vi "populate listbox with logged channels.vi"(7 "MulticolumnListbox in":refnum<vi>, 8 "error in":errorcluster, 11 "Item Ref in":T1 format="%.0x") -> (0 "error out":errorcluster, 2 "logged channel shortnames":string[](array[string]), 3 "logged channel refs":T1[](array[typedef]) format="%.0x")   [LabVIEW 2026, in "Nominal Core Streaming System Explorer.lvlib"]
uses:
  Nominal Core Streaming System Explorer.lvlib
  <vilib>/NI VeriStand/Custom Device API/Custom Device Item Ref.ctl
  <vilib>/NI VeriStand/Custom Device API/Custom Device API.lvlib
  Shared/Nominal Core Streaming Shared.lvlib
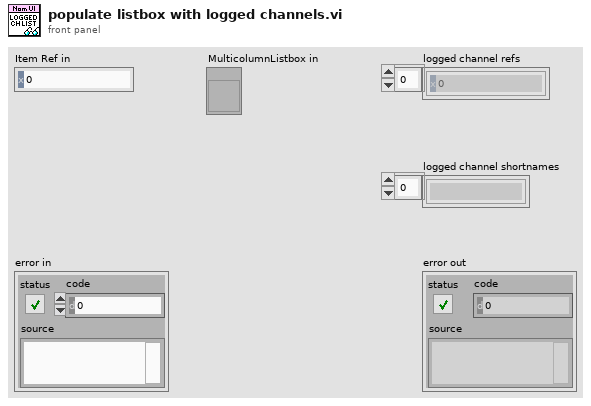
[diagram p1: front panel]
types:
  T1 = typedef "Custom Device API.lvlib/Custom Device Item Ref.ctl" = u64
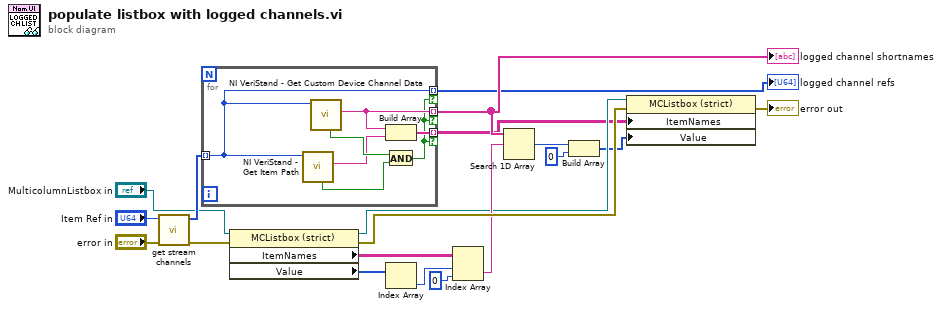
[diagram p0: block diagram]
diagram:
  n1 = call "get stream channels.vi"("error in (no error)"="error in", "Item Ref in"="Item Ref in") -> ("error out"=w4:errorcluster, "Dependent Node Refs"=w18:T1[])  [unwired: 8 in]
  n2 = for {
    tunnel: w18 -> [w21] mode=indexing
    tunnel: [w26] -> w2 mode=indexing if=w20
    tunnel: [w25] -> w3 mode=indexing if=w20
    tunnel: [w21] -> w1 mode=indexing if=w20
    n3 = call <vilib>:"NI VeriStand - Get Item Path.vi"("Item Ref in"=w21) -> ("Path"=w22:string, "Found"=w23:bool)  [unwired: 1 in, 8 out]
    n4 = call <vilib>:"NI VeriStand - Get Custom Device Channel Data.vi"("Channel Ref in"=w21) -> ("Channel Name"=w25:string, "Found"=w24:bool)  [unwired: 5 in, 4 out]
    n5 = Build Array(w25, w22) -> (w26:string[])
    n6 = And(x=w24, y=w23) -> (x .and. y?=w20:bool)
  }
  "logged channel refs" <- w1
  "logged channel shortnames" <- w3
  n7 = property class="MCListbox (strict)"(reference="MulticolumnListbox in", error in=w4) -> (reference out=w8:refnum<vi>, error out=w16:errorcluster, "ItemNames"=w14:string[][], "Value"=w13:i32[])
  n8 = Index Array(array=w13) -> (element=w12:i32)  [unwired: 1 in]
  n9 = Index Array(array=w14, index (row)=w12, index (col)=0 ("disabled index (col)")) -> (element=w10:string)
  n10 = Search 1D Array(1D array=w3, element=w10) -> (index of element=w7:i32)  [unwired: 1 in]
  n11 = Build Array(w7, 0 ("element")) -> (w5:i32[])
  n12 = property class="MCListbox (strict)"(reference=w8, error in=w16, "ItemNames"=w2, "Value"=w5) -> (error out=→"error out":errorcluster)  [unwired: 1 out]
